vi "Comm@Close__Parameter.vi"(1 "ParamterIn":string) -> (0 "ParamterOut":string)   [LabVIEW 2019]
panel:
  in  "CommName":string(combo)
  in  "Confirm":bool
  # "Comm@Close $Comm"
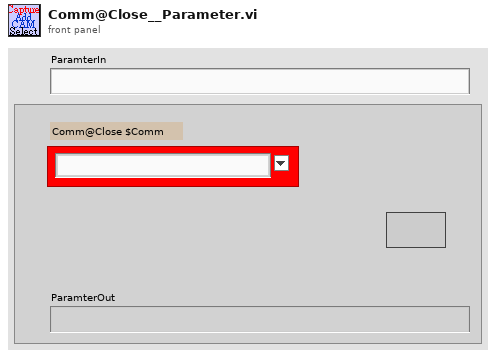
[diagram p1: front panel]
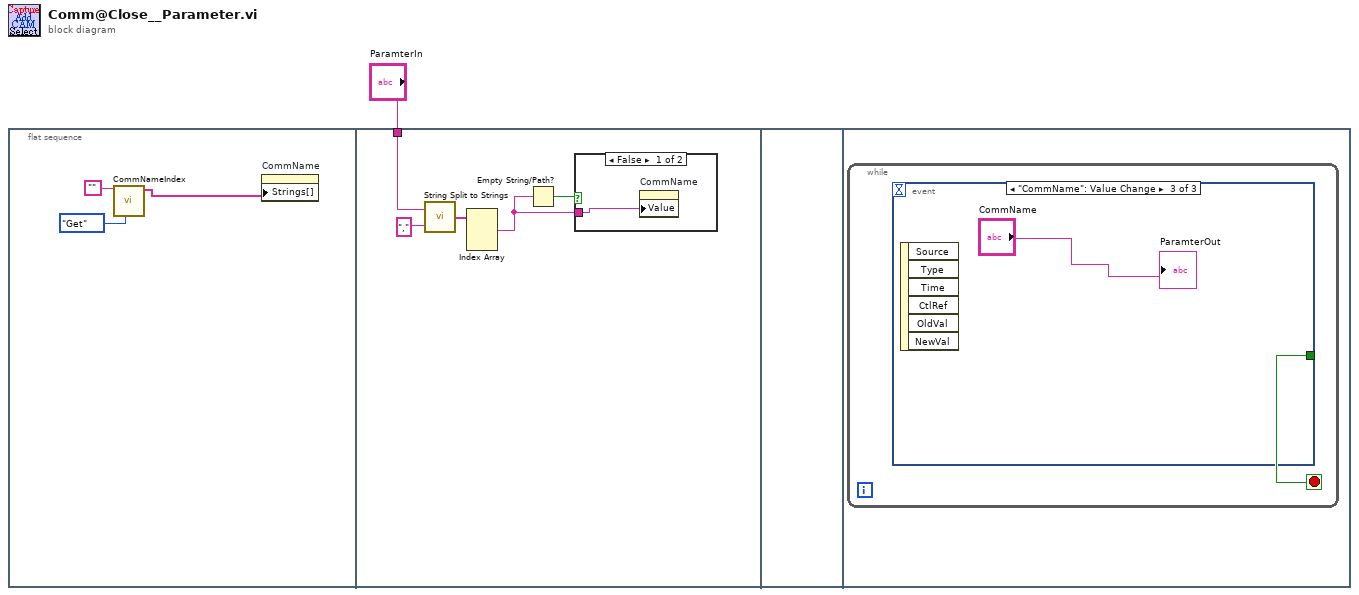
[diagram p0: block diagram]
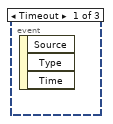
[diagram p3: hidden frame]
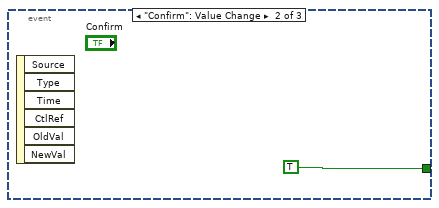
[diagram p4: hidden frame]
diagram:
  n1 = flat-sequence {
    tunnel: "ParamterIn" -> [w7]
    frame #0 {
      n2 = call "CommNameIndex.vi"("OP"=enum16{"Init", "Get", "Set"}."Get", "Comm"="") -> ("CommNameS"=w2:string[])  [unwired: 7 in, 2 out]
      n3 = property on="CommName" class="CmbBox"("Strings[]"=w2) -> ()  [unwired: 2 in, 2 out]
    }
    frame #1 {
      n4 = call "String Split to Strings.vi"("search string/char (-)"=",", "String"=w7) -> ("Array"=w9:string[])
      n5 = Index Array(array=w9) -> (element #1=w5:string)  [unwired: 3 in, 2 out]
      n6 = Empty String/Path?(string/path=w5) -> (empty?=w6:bool)
      n7 = case shown="False" w6 {
        tunnel: w5 -> [w10 _]
        frame False {
          n8 = property on="CommName" class="CmbBox"("Value"=w10) -> ()  [unwired: 2 in, 2 out]
        }
        frame True {
        }
      }
    }
    frame #2 {
    }
    frame #3 {
      n9 = while {
        stop <- w11 stop-if-true
        n10 = event shown="[2] \"CommName\": Value Change" {
          selector: _ -> [_ _ _]
          dyn-events: _ -> [_ _ _]
          timeout: _ -> [_ _ _]
          tunnel: [_ TRUE _] -> w11
          event Timeout {
            n11 = event-data() -> ()  [unwired: 1 in, 3 out]
          }
          event "Confirm": Value Change {
            n12 = event-data() -> ()  [unwired: 1 in, 6 out]
          }
          event "CommName": Value Change {
            n13 = event-data() -> ()  [unwired: 1 in, 6 out]
            "ParamterOut" <- "CommName"
          }
        }
      }
    }
  }
